vi "ConvertDataToTime.vi"(7 "BoardType":u32, 8 "error in (no error)":errorcluster, 9 "Timebase":sgl, 10 "StartTime":dbl, 11 "Data":u32) -> (0 "error out":errorcluster, 3 "ConvertedTime":dbl)   [LabVIEW 2022 SP3, in "EClib functions.lvlib"]
doc: "This VI supplies information on the selected channel."
uses:
  EClib functions.lvlib
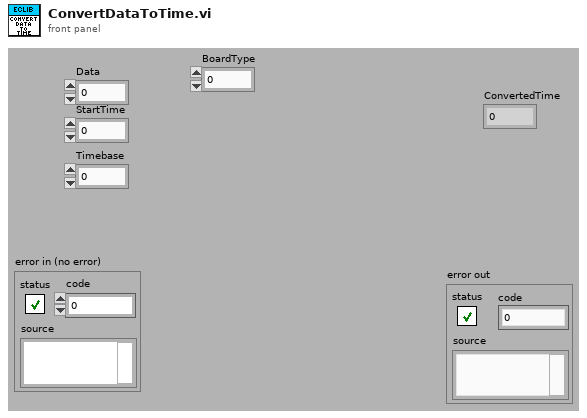
[diagram p1: front panel]
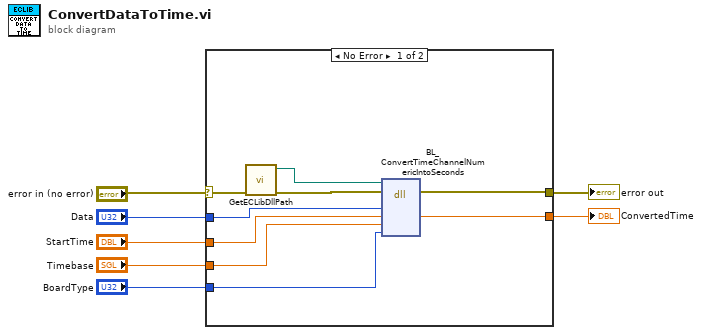
[diagram p0: block diagram]
diagram:
  n1 = case shown="No Error" "error in (no error)" {
    selector: "error in (no error)" -> [w16 w17]
    tunnel: [w13 w17] -> w6
    tunnel: "Data" -> [w12 _]
    tunnel: "StartTime" -> [w11 _]
    tunnel: "Timebase" -> [w10 _]
    tunnel: "BoardType" -> [w9 _]
    tunnel: [w8 _] -> w1
    frame No Error {
      n2 = call "GetECLibDllPath.vi"("error in (no error)"=w16) -> ("error out"=w15:errorcluster, "ECLibDLLPath"=w14:path)  [unwired: 9 in]
      n3 = dll-call lib="?" fn="BL_ConvertTimeChannelNumericIntoSeconds" label="ConvertTime"(path in=w14, error in=w15, "pnum"=w12, "pRetTime"=w11, "Timebase"=w10, "ChannelType"=w9) -> (error out=w13:errorcluster, "pRetTime"=w8:dbl)  [unwired: 5 in, 1 out]
    }
    frame Error {
    }
  }
  "error out" <- w6
  "ConvertedTime" <- w1
